vi "Read Alarm - Message.vi"(8 "error in (no error)":errorcluster, 11 "NT Base in":refnum<class "NT Base.lvclass">) -> (0 "error out":errorcluster, 2 "message":string, 3 "NT Base out":refnum<class "NT Base.lvclass">)   [LabVIEW 2020, in "PV Access.lvlib" / "PV Data.lvlib" / "NT Base.lvclass"]
uses:
  NT Base.lvclass
  NT Base.lvclass/NT Base.ctl
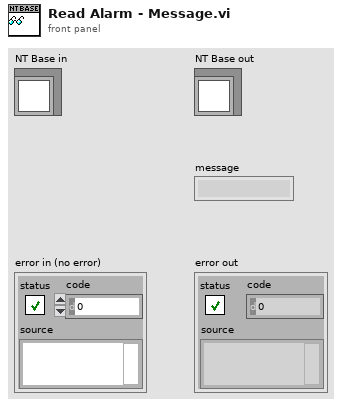
[diagram p1: front panel]
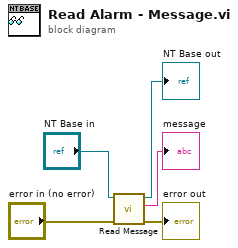
[diagram p0: block diagram]
diagram:
  n1 = call-dynamic "Read Message.vi"("error in"="error in (no error)", "Has Alarm in"="NT Base in") -> ("error out"=→"error out":errorcluster, "message"=→"message":string, "Has Alarm out"=→"NT Base out":refnum<class "NT Base.lvclass">)  [unwired: 7 in]
